vi "TestBench.vi"() -> ()   [LabVIEW 2012]
uses:
  <vilib>/Waveform/DWDTOps.llb/Digital Pattern Generator (Random).vi
  <vilib>/Waveform/DTblOps.llb/DTbl Boolean Array to Digital.vi
panel:
  in  "Data\nSlices":i32
  in  "Slices":u32
  in  "N":i32
  out "Digital Data":digitaldata
  out "Digital Waveform Graph":digitaldata(graph)
  out "Ops/s":dbl
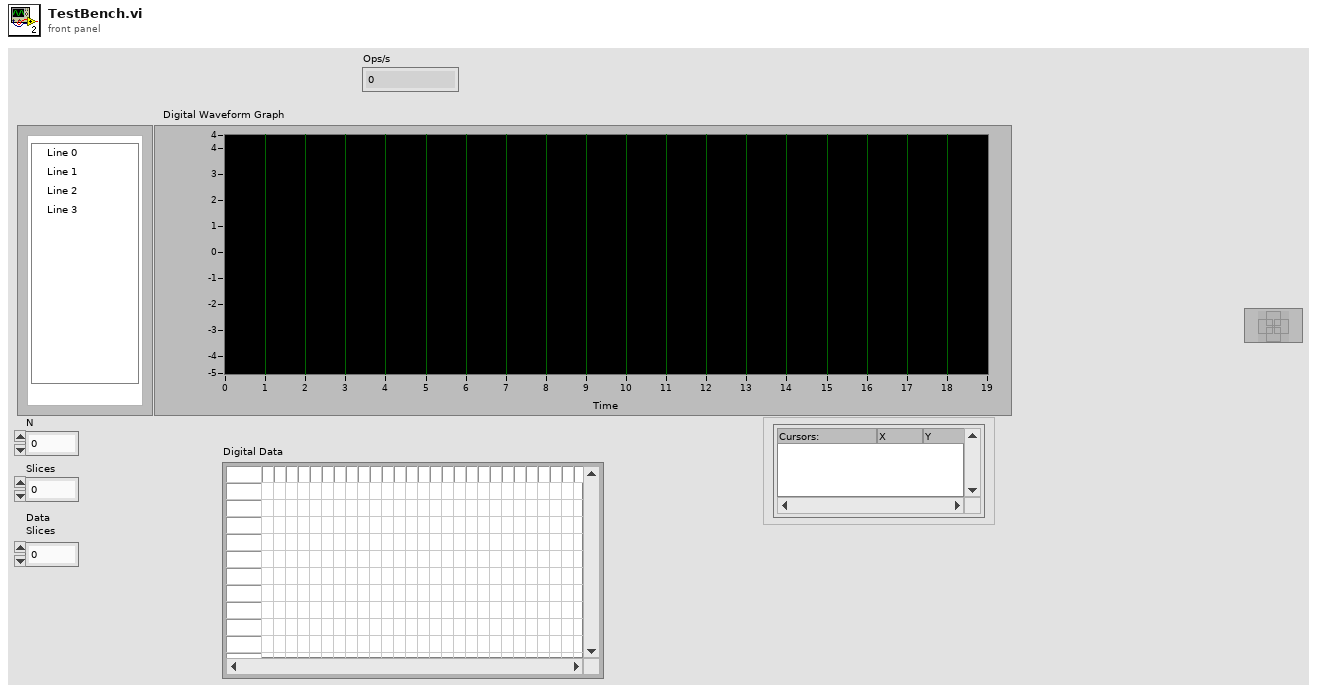
[diagram p1: front panel]
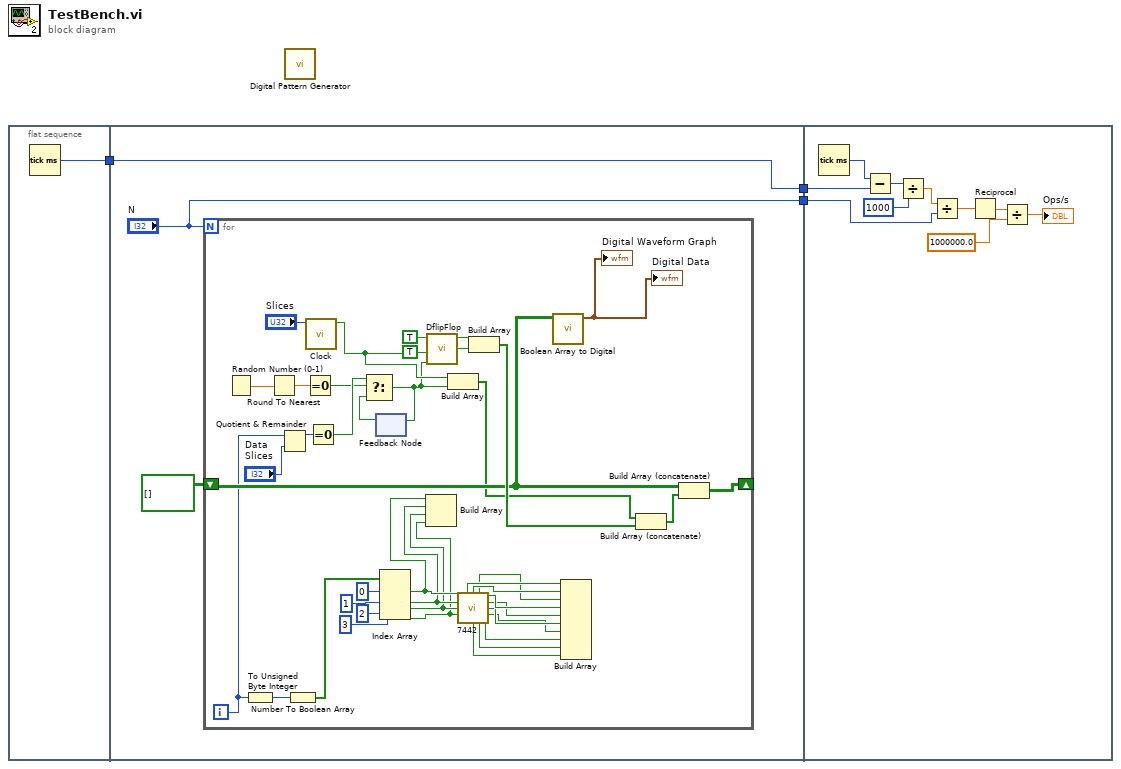
[diagram p0: block diagram]
diagram:
  n1 = flat-sequence {
    tunnel: [w4] -> w2
    tunnel: [w7] -> w3
    tunnel: w2 -> [w7]
    tunnel: ["N"] -> w1
    tunnel: w3 -> [w52]
    tunnel: w1 -> [w55]
    frame #0 {
      n2 = Tick Count (ms)() -> (millisecond timer value=w4:u32)
    }
    frame #1 {
      n3 = for {
        N: "N" -> [_]
        shift-right: [w32] -> _
        shift-left: bool[][] [] -> [w22]
        i -> [w15]
        n4 = Random Number (0-1)() -> (number: 0 to 1=w19:dbl)
        n5 = To Unsigned Byte Integer(number=w15) -> (unsigned 8bit integer=w48:u8)
        n6 = Round To Nearest(number=w19) -> (nearest integer value=w18:dbl)
        n7 = Quotient & Remainder(x=w15, y="Data\nSlices") -> (x-y*floor(x/y)=w14:i32)  [unwired: 1 out]
        n8 = Number To Boolean Array(number=w48) -> (Boolean array=w43:bool[])
        n9 = Equal To 0?(x=w18) -> (x = 0?=w12:bool)
        n10 = call "Clock.vi"("Slices"="Slices") -> ("Clk"=w17:bool)  [unwired: 10 in]
        n11 = Equal To 0?(x=w14) -> (x = 0?=w13:bool)
        n12 = feedback #1() -> (w11:bool)  [unwired: 1 in]
        n13 = Select(t=w12, s=w13, f=w11) -> (s? t:f=w10:bool)
        n14 = feedback-in #1(w10) -> ()
        n15 = Index Array(array=w43, index #1=0 ("index"), index #2=1 ("index"), index #3=2 ("index"), index #4=3 ("index")) -> (element #1=w29:bool, element #2=w28:bool, element #3=w27:bool, element #4=w26:bool)
        n16 = Build Array(w29, w28, w27, w26) -> ()  [unwired: 1 out]
        n17 = call "DflipFlop.vi"("D"=w10, "Clock"=w17, "Reset"=TRUE, "Set"=TRUE) -> ("/Q\\"=w24:bool, "Q"=w25:bool)  [unwired: 6 in]
        n18 = Build Array(w17, w10) -> (w16:bool[])
        n19 = call "7442.vi"("A"=w29, "B"=w28, "C"=w27, "D"=w26) -> ("0"=w42:bool, "1"=w41:bool, "2"=w40:bool, "3"=w39:bool, "4"=w38:bool, "5"=w37:bool, "6"=w36:bool, "9"=w33:bool, "8"=w34:bool, "7"=w35:bool)  [unwired: 2 in]
        n20 = Build Array(w25, w24) -> (w23:bool[])
        n21 = call-poly <vilib>:"Boolean Array to Digital.vi"("boolean array"=w22) -> ("digital data"=→"Digital Waveform Graph" →"Digital Data":digitaldata)  [unwired: 9 in, 1 out]
        n22 = Build Array(w42, w41, w40, w39, w38, w37, w36, w35, w34, w33) -> ()  [unwired: 1 out]
        n23 = Build Array (concatenate)(w16, w23) -> (w31:bool[])
        n24 = Build Array (concatenate)(w22, w31) -> (w32:bool[][])
      }
    }
    frame #2 {
      n25 = Tick Count (ms)() -> (millisecond timer value=w53:u32)
      n26 = Subtract(x=w53, y=w52) -> (x-y=w58:u32)
      n27 = Divide(x=w58, y=u16 1000) -> (x/y=w56:dbl)
      n28 = Divide(x=w56, y=w55) -> (x/y=w54:dbl)
      n29 = Reciprocal(x=w54) -> (1/x=w51:dbl)
      n30 = Divide(x=w51, y=1000000.0) -> (x/y=→"Ops/s":dbl)
    }
  }
  n31 = call-poly <vilib>:"Digital Pattern Generator.vi"() -> ()  [unwired: 10 in, 2 out]
